vi "Load_Traverse_file.vi"(0 "Setup filename":path) -> (3 "Setup filename Out":path, 4 "Jump Bad Positions":bool, 5 "Table":T2[](array[typedef]) {"Carrier_2 Q (l/min)" format="%#.2f"; "Row Duration (mins)" format="%#.1f"; "Row No" min=0; "Trace Gas Concentration (%)" min=0.0 format="%#_4f"; "Carrier_1 Q (l/min)" format="%#.2f"; "Tunnel Speed" format="%#.2f"; "Start X" format="%#.2f"; "Start Y" format="%#.2f"; "Start Z" format="%#.2f"; "End X" format="%#.2f"; "End Y" format="%#.2f"; "End Z" format="%#.2f"; "Averaging time (min)" min=0.0 format="%#.2f"}, 6 "Work in Tunnel Coordinates?":T1)   [LabVIEW 2014]
uses:
  Traverse_cluster.ctl
  Spacing.ctl
  Controls/Multi_run_mode.ctl
  Controls/Tunnel_Coordinates.ctl
panel:
  # "HD:Users"
  # "HD:Users"
  # "X           Y            Z"
  # "Start"
  # "End"
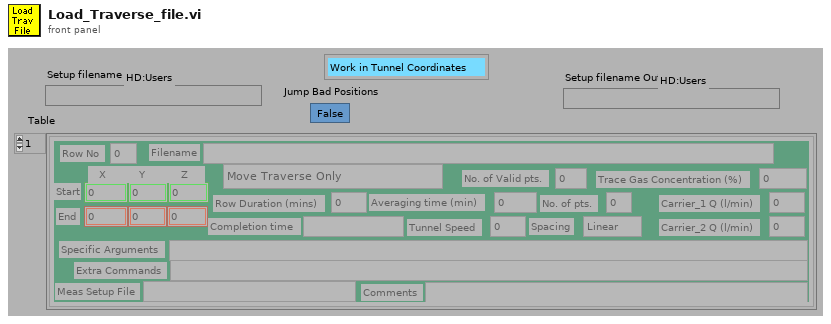
[diagram p1: front panel]
types:
  T1 = typedef "Tunnel_Coordinates.ctl" = enum16{"Work in Tunnel Coordinates", "Work in Model Coordinates"}
  T2 = typedef "Traverse_cluster.ctl" = cluster{"Start X":sgl, "Start Y":sgl, "Start Z":sgl, "End X":sgl, "End Y":sgl, "End Z":sgl, "No. of pts.":i32, "Spacing":T3, "Filename":path, "Tunnel Speed":dbl, "Averaging time (min)":dbl, "Extra Commands":string, "Carrier_1 Q (l/min)":dbl, "Carrier_2 Q (l/min)":dbl, "Trace Gas Concentration (%)":dbl, "Specific Arguments":string, "Comments":string, "Row No":i32, "Row Type Selector":T4, "Completion time":string, "Row Duration (mins)":dbl, "No. of Valid pts.":i32, "Meas Setup File":string}
  T3 = typedef "Spacing.ctl" = enum16{"Linear", "Log", "Gauss", "Specified", "N/A"}
  T4 = typedef "Multi_run_mode.ctl" = enum16{"Move Traverse Only", "Set Tunnel Speed Only", "Set Source Only", "Set Measurement Conditions", "Single Measurement", "Vertical Profile", "Lateral Profile", "Longitudinal Profile", "Explore Volume", "Multi-Axis Profile", "Auto Calibrate", "Meas Fast FID Bkgnd", "Check Beam Power", "Scanning Valve Measurement", "Run VI Named:", "Set ADAM Ch", "Wait (minutes)", "Send Message", "Synchronize With:", "Fall Back to this Row", "Turn Off Row Repeating", "Blank Row", "Traverse 3D Volume"}
  T5 = enum16{"All Channel Names", "Valid Channel Names"}
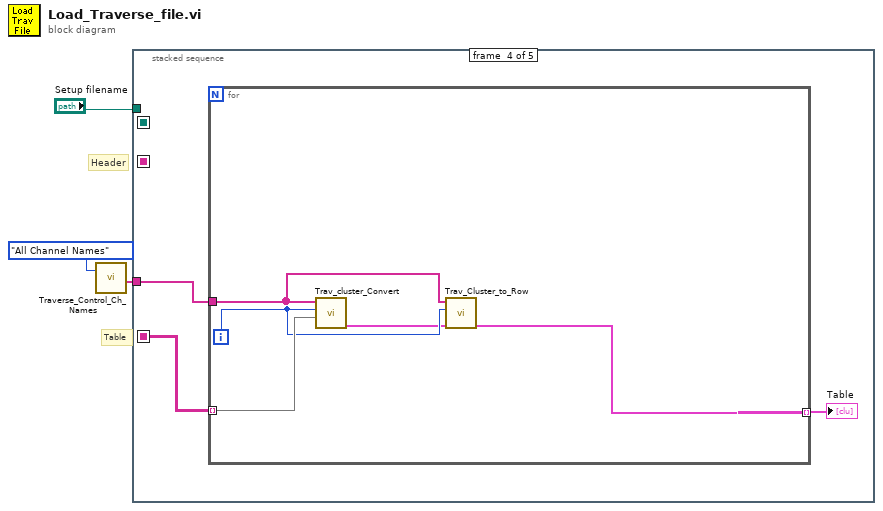
[diagram p0: block diagram]
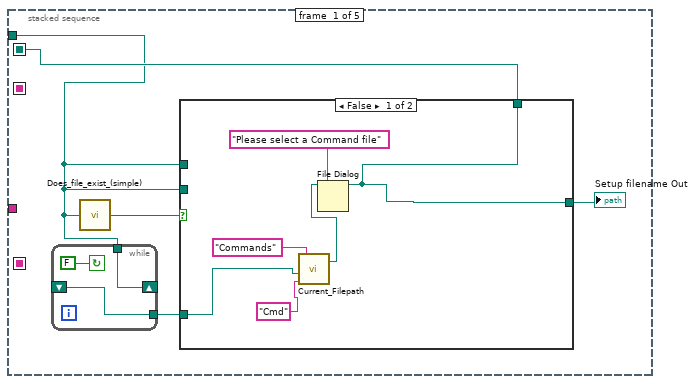
[diagram p2: hidden frame]
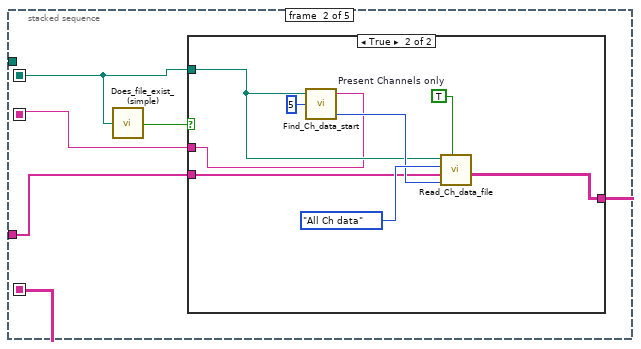
[diagram p4: hidden frame]
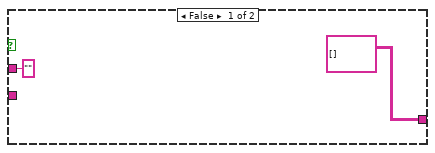
[diagram p5: hidden frame]
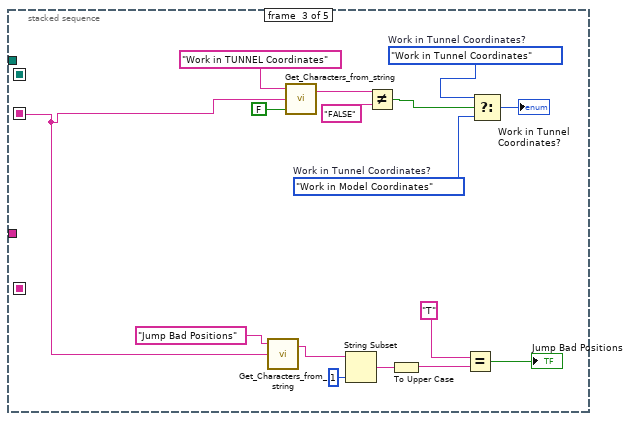
[diagram p6: hidden frame]
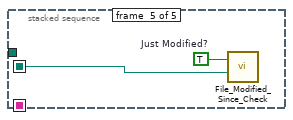
[diagram p7: hidden frame]
diagram:
  # "Header"
  # "Table"
  n1 = call "Traverse_Control_Ch_Names.vi"("Mode"=T5."All Channel Names") -> ("Channel names"=w2:string[])  [unwired: 1 in]
  n2 = stacked-sequence {
    seq-local: [_ w24 _ _ _] -> [_ _ _ w53 _]
    seq-local: [_ w23 _ _ _] -> [_ _ w41 _ _]
    seq-local: [w8 _ _ _ _] -> [_ w21 _ _ w59]
    tunnel: "Setup filename" -> [w4 _ _ _ _]
    tunnel: w2 -> [_ w20 _ w52 _]
    frame #0 {
      n3 = while {
        tunnel: [w10] -> w5
        tunnel: w4 -> [w11]
        shift-left: _ -> [w10]
        shift-right: [w11] -> _
        stop <- FALSE continue-if-true
      }
      n4 = call "Does_file_exist_(simple).vi"("Pathname"=w4) -> ("exists?"=w6:bool)
      n5 = case shown="False" w6 {
        tunnel: w4 -> [_ w19]
        tunnel: [w16 w19] -> w8
        tunnel: [w16 w18] -> w7
        tunnel: w4 -> [_ w18]
        tunnel: w5 -> [w14 _]
        frame False {
          n6 = call "Current_Filepath.vi"("Short_Name"="Cmd" ("Data Type"), "Filename in"=w14, "Data Type"="Commands") -> ("Directory"=w13:path)  [unwired: 1 in, 1 out]
          n7 = File Dialog(7:"Please select a Command file" ("prompt"), 11:w13) -> (3:w16:path)  [unwired: 1 in, 7 out]
        }
        frame True {
        }
      }
      "Setup filename Out" <- w7
    }
    frame #1 {
      n8 = call "Does_file_exist_(simple).vi"("Pathname"=w21) -> ("exists?"=w22:bool)
      n9 = case shown="True" w22 {
        tunnel: [string[][] [] w29] -> w24
        tunnel: ["" ("character string") w30] -> w23
        tunnel: w21 -> [_ w31]
        tunnel: w20 -> [_ w28]
        frame False {
        }
        frame True {
          w34 = TRUE  # Present Channels only
          n10 = call "Find_Ch_data_start.vi"("Approx No Of Columns"=5, "Filename"=w31) -> ("Start of read offset output"=w32:i32, "String before data"=w30:string)  [unwired: 1 in, 1 out]
          n11 = call "Read_Ch_data_file.vi"("Present Channels only"=w34, "Start of read offset (chars.: 0)"=w32, "Present Channels"=w28, "Output"=enum16{"All Ch data", "The last few rows"}."All Ch data", "Filename"=w31) -> ("Channel Values"=w29:string[][])  [unwired: 4 out]
        }
      }
    }
    frame #2 {
      w44 = Tunnel_Coordinates."Work in Model Coordinates"  # Work in Tunnel Coordinates?
      w46 = Tunnel_Coordinates."Work in Tunnel Coordinates"  # Work in Tunnel Coordinates?
      n12 = call "Get_Characters_from_string.vi"("Input string"=w41, "Variable name"="Jump Bad Positions" ("Label for characters")) -> ("Value"=w36:string)  [unwired: 1 in, 1 out]
      n13 = call "Get_Characters_from_string.vi"("Show Dialog?"=FALSE, "Input string"=w41, "Variable name"="Work in TUNNEL Coordinates" ("Label for characters")) -> ("Value"=w49:string)  [unwired: 1 out]
      n14 = String Subset(string=w36, length (rest)=1 ("length")) -> (substring=w38:string)  [unwired: 1 out]
      n15 = Not Equal?(x=w49, y="FALSE") -> (x != y?=w47:bool)
      n16 = To Upper Case(1:w38) -> (0:w37:string)
      n17 = Equal?(x="T", y=w37) -> (x = y?=→"Jump Bad Positions":bool)
      n18 = Select(t=w46, s=w47, f=w44) -> (s? t:f=→"Work in Tunnel Coordinates?":T1)
    }
    frame #3 {
      n19 = for {
        tunnel: w53 -> [w58] mode=indexing
        tunnel: [w55] -> w51 mode=indexing
        tunnel: w52 -> [w57]
        i -> [w56]
        n20 = call "Trav_cluster_Convert.vi"("Channel Values In"=w58, "Row Number"=w56, "Channel names"=w57) -> ("Traverse line Out"=w54:T2)  [unwired: 1 in, 3 out]
        n21 = call "Trav_Cluster_to_Row.vi"("Traverse line in"=w54, "Row Number"=w56, "Channel names"=w57) -> ("Traverse line Out"=w55:T2)  [unwired: 4 out]
      }
      "Table" <- w51
    }
    frame #4 {
      w60 = TRUE  # Just Modified?
      n22 = call "File_Modified_Since_Check.vi"("Pathname"=w59, "Just Modified?"=w60) -> ()  [unwired: 1 out]
    }
  }
